vi "Generate_WayPoints_Hopping_CV.vi"(8 "NumberOfCVsAtEachPoint":i32=1, 11 "Input Cluster":T2={"Scan Rate (um/s)"=15.0, "X Start"=15.0, "X End"=15.0, "Y Start"=15.0, "Y End"=15.0, " Z Start"=15.0, "HoppingDistance"=1.0, "V"=15.0, "Z End"=15.0, "Approach Rate Hopping (um/s)"=15.0, "Retrack Rate (um/s)"=15.0, "V 2"=15.0, "Approach Rate (um/s)"=15.0, "V 3"=15.0, "CV Rate / V/s"=15.0, "V 4"=15.0, "V 1"=15.0, "HoldTime1/s"=15.0, "Hold time 2 / s"=15.0, "Hold time 3/ s"=15.0, "HoppingDistanceBetweenLines"=1.0}) -> (0 "output cluster":T1, 3 "WaitTimeScaler":u64)   [LabVIEW 2023]
uses:
  TypeDefs/WayPointCluster.ctl
  TypeDefsControls/Time.ctl
  User_Vi/Settings.vi
panel:
  in  "WayPointCluster 2":T1
  out "Y  P":dbl
  out "X  P":dbl
  out "HoppingDistanceX":dbl
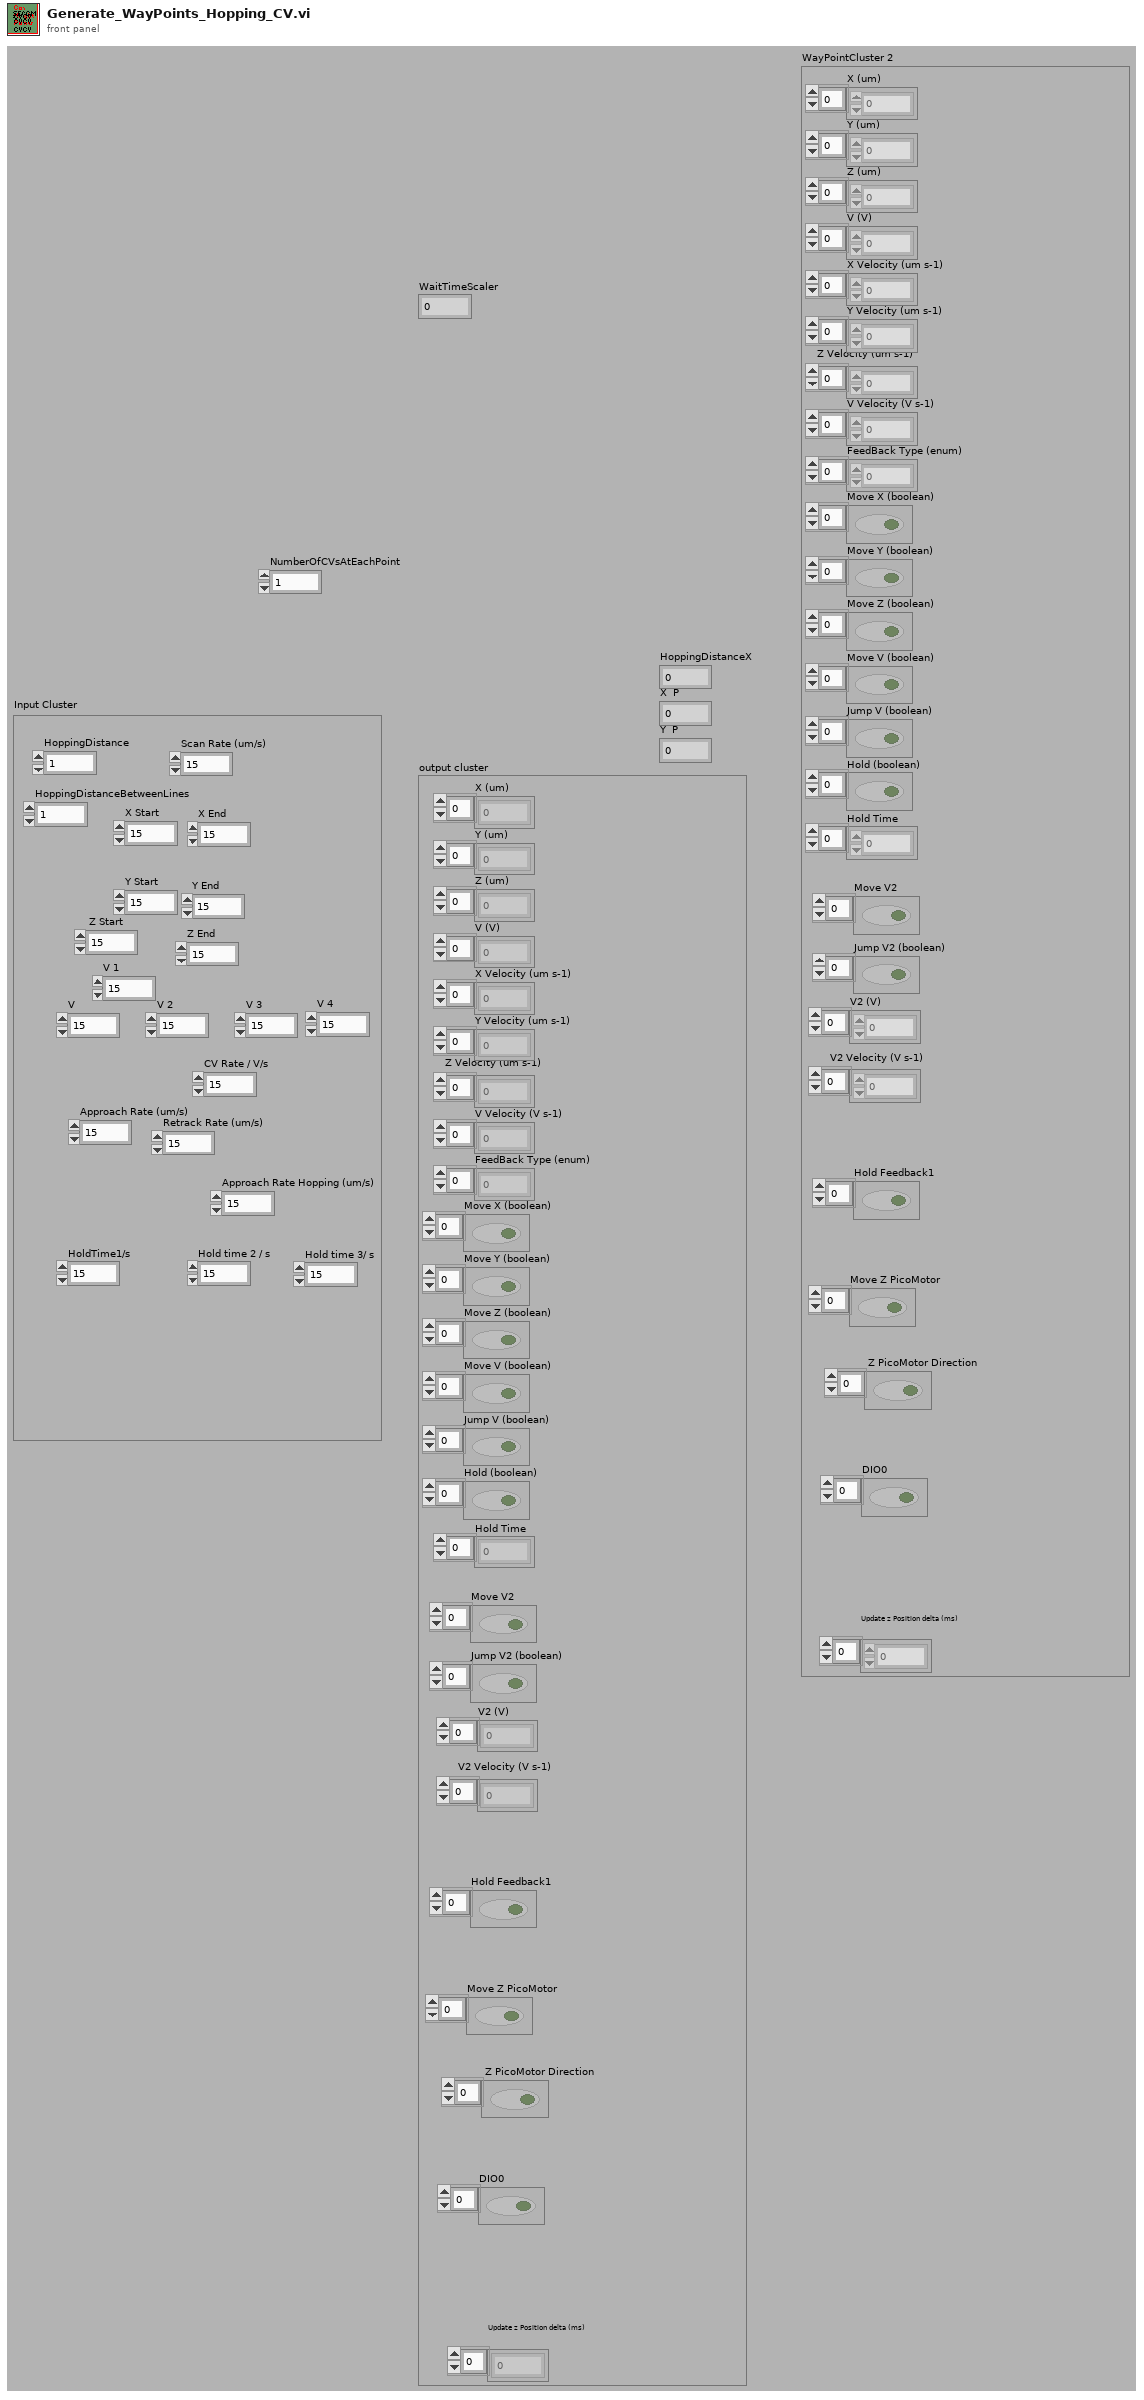
[diagram p1: front panel]
types:
  T1 = typedef "WayPointCluster.ctl" = cluster{"X (um)":dbl[], "Y (um)":dbl[], "Z (um)":dbl[], "V (V)":dbl[], "X Velocity (um s-1)":dbl[], "Y Velocity (um s-1)":dbl[], "Z Velocity (um s-1)":dbl[], "V Velocity (V s-1)":dbl[], "FeedBack Type (enum)":u16[], "Move X (boolean)":bool[], "Move Y (boolean)":bool[], "Move Z (boolean)":bool[], "Move V (boolean)":bool[], "Jump V (boolean)":bool[], "Hold (boolean)":bool[], "Hold Time":u32[], "V2 (V)":dbl[], "Move V2":bool[], "V2 Velocity (V s-1)":dbl[], "Jump V2 (boolean)":bool[], "Update z Position delta (ms)":i16[], "Hold Feedback1":bool[], "Move Z PicoMotor":bool[], " Z PicoMotor Direction":bool[], "DIO0":bool[]}
  T2 = cluster{"Scan Rate (um/s)":dbl, "X Start":dbl, "X End":dbl, "Y Start":dbl, "Y End":dbl, " Z Start":dbl, "HoppingDistance":dbl, "V":dbl, "Z End":dbl, "Approach Rate Hopping (um/s)":dbl, "Retrack Rate (um/s)":dbl, "V 2":dbl, "Approach Rate (um/s)":dbl, "V 3":dbl, "CV Rate / V/s":dbl, "V 4":dbl, "V 1":dbl, "HoldTime1/s":dbl, "Hold time 2 / s":dbl, "Hold time 3/ s":dbl, "HoppingDistanceBetweenLines":dbl}
  T3 = typedef "Time.ctl" = dbl
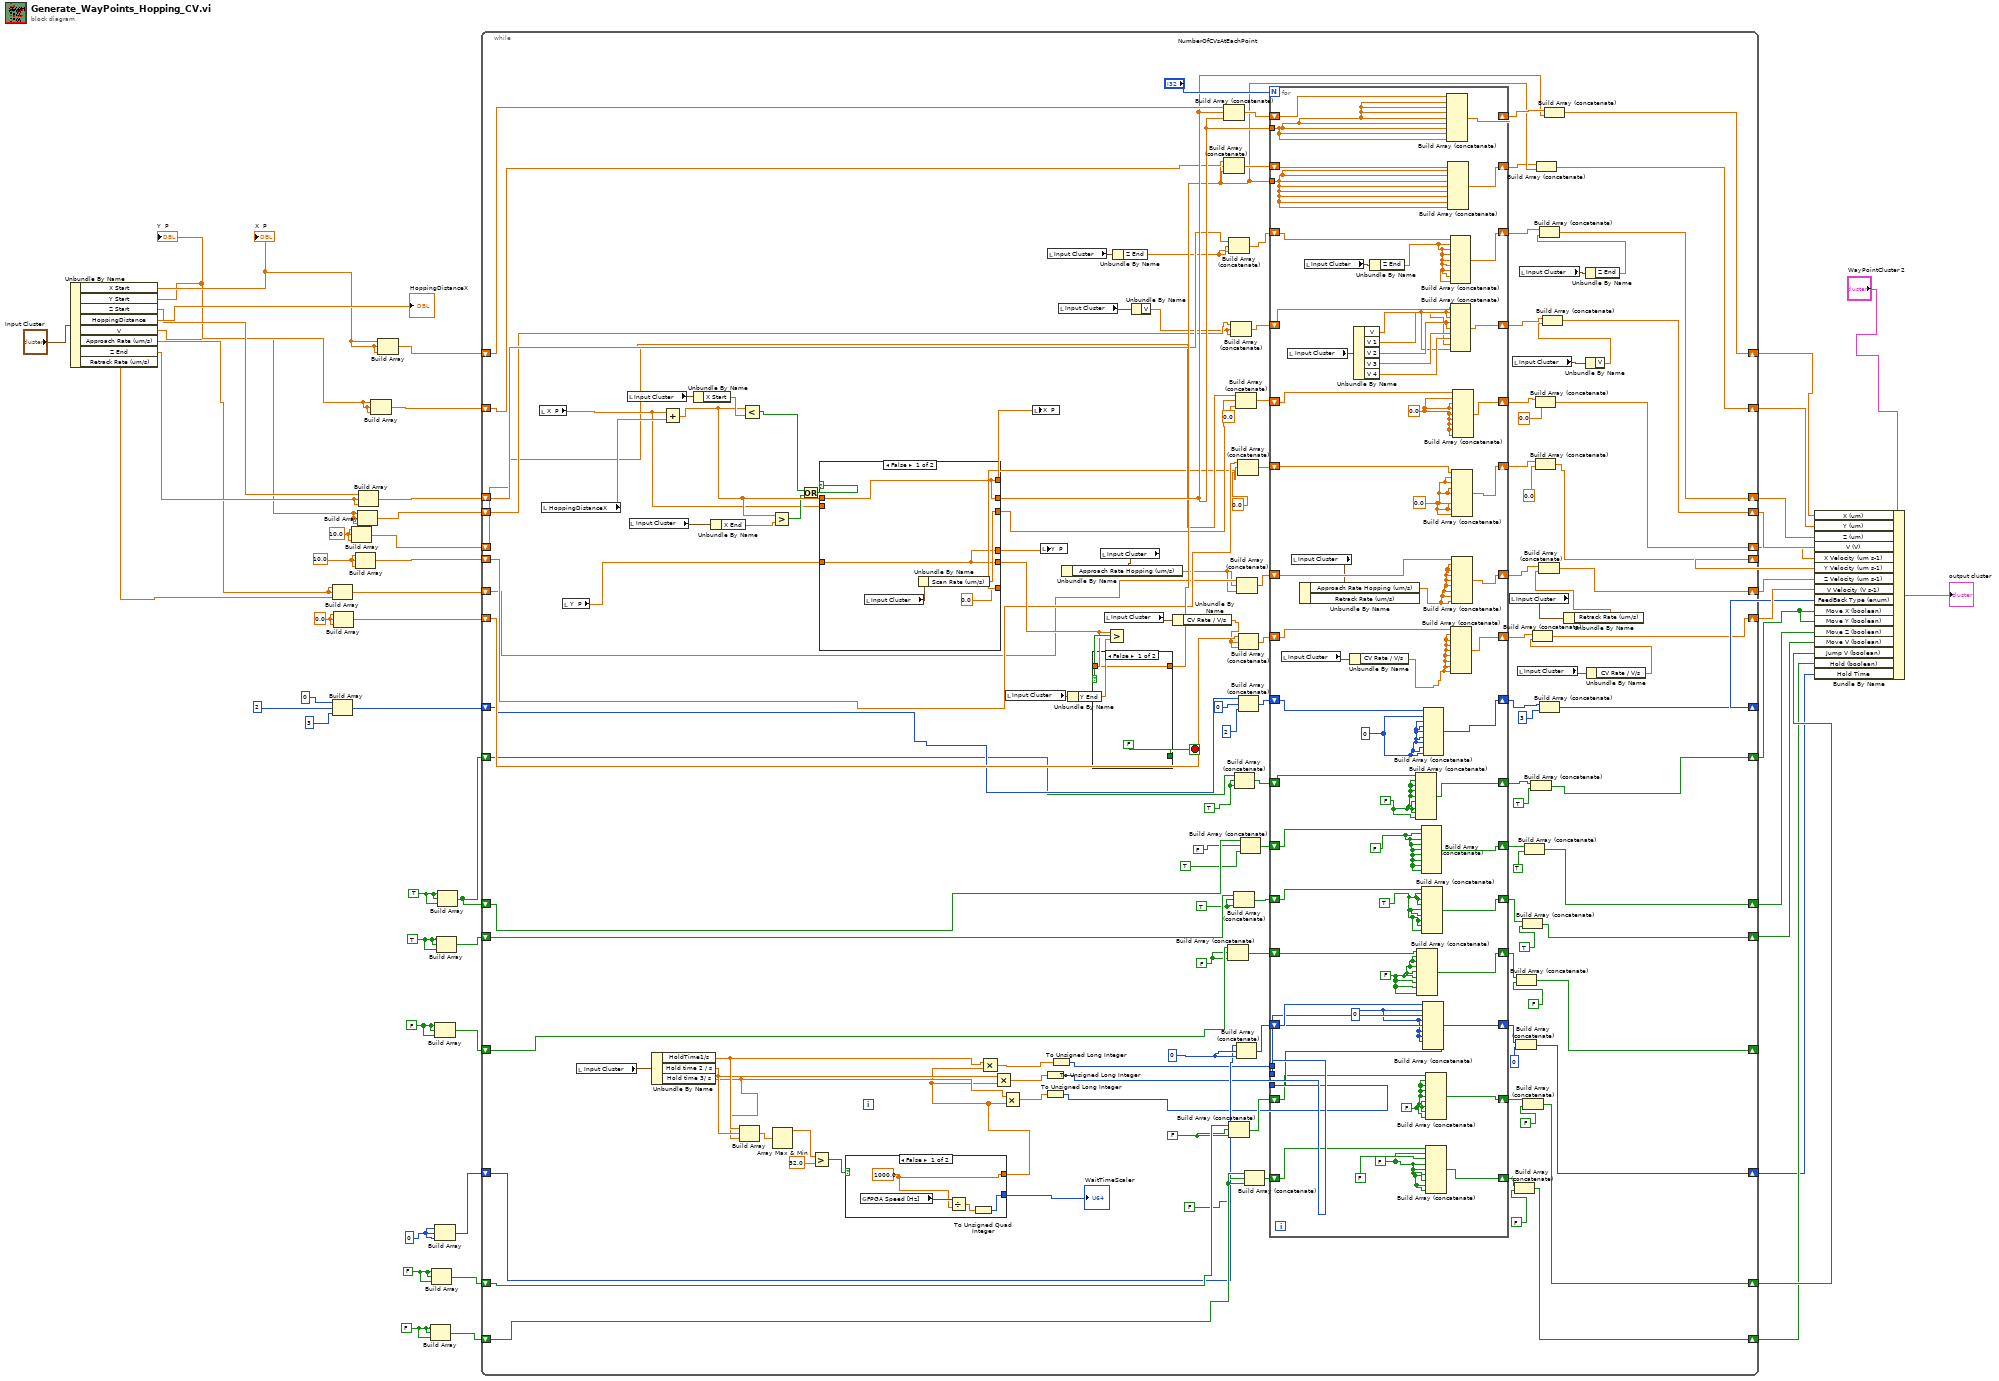
[diagram p0: block diagram]
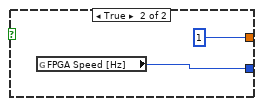
[diagram p2: hidden frame]
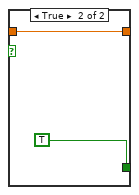
[diagram p3: hidden frame]
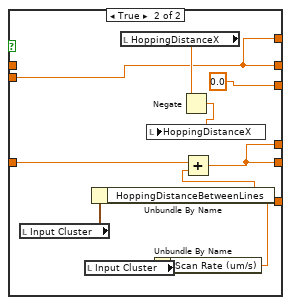
[diagram p4: hidden frame]
diagram:
  w10 = FALSE
  w18 = FALSE
  w22 = FALSE
  w21 = u32 0 ("element")
  w20 = TRUE
  w16 = TRUE
  w12 = 10.0 ("element")
  w13 = 10.0 ("element")
  w15 = 0.0 ("element")
  n1 = Unbundle By Name("Input Cluster") -> ("X Start"=w34:dbl, "Y Start"=w33:dbl, "Z Start"=w35:dbl, "HoppingDistance"=→"HoppingDistanceX":dbl, "V"=w31:dbl, "Approach Rate (um/s)"=w14:dbl, "Z End"=w32:dbl, "Retrack Rate (um/s)"=w30:dbl)
  "X  P" <- w34
  "Y  P" <- w33
  n2 = Build Array(w14, w14, w30) -> (w42:dbl[])
  n3 = Build Array(u16 0 ("element"), u16 2 ("element"), u16 3 ("element")) -> (w38:u16[])
  n4 = Build Array(w15, w15, w15) -> (w40:dbl[])
  n5 = Build Array(w12, w12, w12) -> (w45:dbl[])
  n6 = Build Array(w13, w13, w13) -> (w44:dbl[])
  n7 = Build Array(w31, w31, w31) -> (w47:dbl[])
  n8 = Build Array(w35, w32, w32) -> (w49:dbl[])
  n9 = Build Array(w33, w33, w33) -> (w50:dbl[])
  n10 = Build Array(w34, w34, w34) -> (w51:dbl[])
  n11 = Build Array(w10, w10, w10) -> (w9:bool[])
  n12 = Build Array(w22, w22, w22) -> (w26:bool[])
  n13 = Build Array(w18, w18, w18) -> (w17:bool[])
  n14 = Build Array(w21, w21, w21) -> (w4:u32[])
  n15 = Build Array(w20, w20, w20) -> (w24:bool[])
  n16 = Build Array(w16, w16, w16) -> (w11:bool[])
  n17 = while {
    shift-right: [w171] -> w6
    shift-left: w51 -> [w174]
    shift-right: [w165] -> w5
    shift-left: w50 -> [w169]
    shift-right: [w159] -> w48
    shift-left: w49 -> [w164]
    shift-right: [w155] -> w46
    shift-left: w47 -> [w153]
    shift-right: [w143] -> w28
    shift-left: w45 -> [w148]
    shift-right: [w135] -> w43
    shift-left: w44 -> [w141]
    shift-right: [w129] -> w41
    shift-left: w42 -> [w134]
    shift-right: [w120] -> w39
    shift-left: w40 -> [w126]
    shift-right: [w114] -> w37
    shift-left: w38 -> [w112]
    shift-right: [w102] -> w27
    shift-left: w11 -> [w105]
    shift-right: [w89] -> _
    shift-left: w17 -> [w92]
    shift-right: [w79] -> w25
    shift-left: w26 -> [w82]
    shift-right: [w95] -> w19
    shift-left: w24 -> [w98]
    shift-right: [w107] -> w7
    shift-left: w11 -> [w111]
    shift-right: [w75] -> w8
    shift-left: w9 -> [w78]
    shift-right: [w63] -> w3
    shift-left: w4 -> [w70]
    stop <- w182 stop-if-true
    w72 = FALSE
    w74 = FALSE
    w84 = u32 0 ("element")
    w88 = FALSE
    w93 = TRUE
    w109 = TRUE
    n18 = local read "X  P"() -> (w181:dbl)
    n19 = local read "HoppingDistanceX"() -> (w192:dbl)
    n20 = local read "Y  P"() -> (w180:dbl)
    n21 = local read "Input Cluster"() -> (w176:T2)
    n22 = local read "Input Cluster"() -> (w194:T2)
    n23 = local read "Input Cluster"() -> (w193:T2)
    n24 = Unbundle By Name(w176) -> ("HoldTime1/s"=w62:dbl, "Hold time 2 / s"=w61:dbl, "Hold time 3/ s"=w60:dbl)
    n25 = Add(x=w181, y=w192) -> (x+y=w188:dbl)
    n26 = Unbundle By Name(w194) -> ("X Start"=w191:dbl)
    n27 = Unbundle By Name(w193) -> ("X End"=w189:dbl)
    n28 = Build Array(w62, w61, w60) -> (w59:dbl[])
    n29 = Less?(x=w188, y=w191) -> (x < y?=w190:bool)
    n30 = Greater?(x=w188, y=w189) -> (0:w187:bool)
    n31 = Array Max & Min(array=w59) -> (max value=w57:dbl)  [unwired: 3 out]
    n32 = Or(x=w190, y=w187) -> (x .or. y?=w186:bool)
    n33 = Greater?(x=w57, y=T3 32.0) -> (0:w56:bool)
    n34 = case shown="False" w186 {
      tunnel: w188 -> [w265 _]
      tunnel: [w265 w271] -> w170
      tunnel: w181 -> [_ w271]
      tunnel: w180 -> [w266 w272]
      tunnel: [w266 w270] -> w179
      tunnel: [w268 0.0] -> w146
      tunnel: [0.0 w273] -> w139
      tunnel: [w266 w270] -> w178
      tunnel: [w265 w271] -> w177
      frame False {
        n35 = local read "Input Cluster"() -> (w269:T2)
        n36 = Unbundle By Name(w269) -> ("Scan Rate (um/s)"=w268:dbl)
      }
      frame True {
        n37 = local read "Input Cluster"() -> (w277:T2)
        n38 = local read "Input Cluster"() -> (w275:T2)
        n39 = Unbundle By Name(w277) -> ("HoppingDistanceBetweenLines"=w276:dbl)
        n40 = local read "HoppingDistanceX"() -> (w279:dbl)
        n41 = Unbundle By Name(w275) -> ("Scan Rate (um/s)"=w273:dbl)
        n42 = Negate(x=w279) -> (-x=w278:dbl)
        n43 = local write "HoppingDistanceX"(w278) -> ()
        n44 = Add(x=w272, y=w276) -> (x+y=w270:dbl)
      }
    }
    n45 = case shown="False" w56 {
      tunnel: [w196 w200] -> w55
      tunnel: [w195 1] -> w54
      frame False {
        w195 = 1000.0 ("y")
        n46 = global read "Settings.vi" "FPGA Speed [Hz]"() -> (w198:i64)
        n47 = Divide(x=w198, y=w195) -> (x/y=w197:dbl)
        n48 = To Unsigned Quad Integer(1:w197) -> (0:w196:u64)
      }
      frame True {
        n49 = global read "Settings.vi" "FPGA Speed [Hz]"() -> (w200:i64)
      }
    }
    "WaitTimeScaler" <- w55
    n50 = Multiply(x=w62, y=w54) -> (x*y=w69:dbl)
    n51 = Multiply(x=w61, y=w54) -> (x*y=w67:dbl)
    n52 = Multiply(x=w60, y=w54) -> (x*y=w65:dbl)
    n53 = local read "Input Cluster"() -> (w185:T2)
    n54 = local write "X  P"(w177) -> ()
    n55 = local write "Y  P"(w178) -> ()
    n56 = To Unsigned Long Integer(number=w65) -> (unsigned 32bit integer=w64:u32)
    n57 = To Unsigned Long Integer(number=w67) -> (unsigned 32bit integer=w66:u32)
    n58 = local read "Input Cluster"() -> (w163:T2)
    n59 = To Unsigned Long Integer(number=w69) -> (unsigned 32bit integer=w68:u32)
    n60 = local read "Input Cluster"() -> (w154:T2)
    n61 = Unbundle By Name(w185) -> ("Y End"=w184:dbl)
    n62 = local read "Input Cluster"() -> (w132:T2)
    n63 = Unbundle By Name(w132) -> ("Approach Rate Hopping (um/s)"=w131:dbl)
    n64 = local read "Input Cluster"() -> (w124:T2)
    n65 = Greater?(x=w179, y=w184) -> (0:w183:bool)
    n66 = case shown="False" w183 {
      tunnel: w179 -> [w262 w264]
      tunnel: [w262 w264] -> w167
      tunnel: [FALSE TRUE] -> w182
      frame False {
      }
      frame True {
      }
    }
    n67 = Unbundle By Name(w163) -> ("Z End"=w162:dbl)
    n68 = Unbundle By Name(w154) -> ("V"=w151:dbl)
    n69 = Unbundle By Name(w124) -> ("CV Rate / V/s"=w123:dbl)
    n70 = Build Array (concatenate)(w174, w170, w170) -> (w173:dbl[])
    n71 = Build Array (concatenate)(w169, w167, w167) -> (w168:dbl[])
    n72 = Build Array (concatenate)(w92, w88, w88) -> (w91:bool[])
    n73 = Build Array (concatenate)(w164, w162, w162) -> (w161:dbl[])
    n74 = Build Array (concatenate)(w82, w74, w74) -> (w81:bool[])
    n75 = Build Array (concatenate)(w153, w151, w151) -> (w152:dbl[])
    n76 = Build Array (concatenate)(w98, w93, w93) -> (w97:bool[])
    n77 = Build Array (concatenate)(w111, w109, w109) -> (w110:bool[])
    n78 = Build Array (concatenate)(w148, w146, 0.0 ("element")) -> (w147:dbl[])
    n79 = Build Array (concatenate)(w70, w84, w84) -> (w86:u32[])
    n80 = Build Array (concatenate)(w134, w131, w131) -> (w133:dbl[])
    n81 = Build Array (concatenate)(w141, w139, 0.0 ("element")) -> (w140:dbl[])
    n82 = Build Array (concatenate)(w126, w123, w123) -> (w125:dbl[])
    n83 = Build Array (concatenate)(w112, u16 0 ("element"), u16 2 ("element")) -> (w118:u16[])
    n84 = Build Array (concatenate)(w105, FALSE, TRUE) -> (w104:bool[])
    n85 = Build Array (concatenate)(w78, w72, w72) -> (w77:bool[])
    n86 = for {
      N: "NumberOfCVsAtEachPoint" -> [_]
      shift-right: [w259] -> w172
      shift-left: w173 -> [w260]
      tunnel: w170 -> [w258]
      shift-right: [w255] -> w166
      shift-left: w168 -> [w257]
      tunnel: w167 -> [w256]
      shift-right: [w251] -> w160
      shift-left: w161 -> [w254]
      shift-right: [w249] -> w156
      shift-left: w152 -> [w250]
      shift-right: [w240] -> w144
      shift-left: w147 -> [w242]
      shift-right: [w238] -> w137
      shift-left: w140 -> [w239]
      shift-right: [w235] -> w130
      shift-left: w133 -> [w236]
      shift-right: [w232] -> w121
      shift-left: w125 -> [w231]
      shift-right: [w227] -> w115
      shift-left: w118 -> [w228]
      shift-right: [w224] -> w108
      shift-left: w110 -> [w225]
      shift-right: [w221] -> w103
      shift-left: w104 -> [w222]
      shift-right: [w218] -> w96
      shift-left: w97 -> [w219]
      shift-right: [w215] -> w90
      shift-left: w91 -> [w216]
      shift-right: [w212] -> w85
      shift-left: w86 -> [w213]
      tunnel: w68 -> [w211]
      tunnel: w66 -> [w210]
      tunnel: w64 -> [w208]
      shift-right: [w206] -> w80
      shift-left: w81 -> [w207]
      shift-right: [w204] -> w76
      shift-left: w77 -> [w205]
      w201 = FALSE
      w203 = FALSE
      w209 = u32 0 ("element")
      w214 = FALSE
      w217 = TRUE
      w220 = FALSE
      w223 = FALSE
      w226 = u16 0 ("element")
      w237 = 0.0 ("element")
      w241 = 0.0 ("element")
      n87 = local read "Input Cluster"() -> (w230:T2)
      n88 = local read "Input Cluster"() -> (w248:T2)
      n89 = local read "Input Cluster"() -> (w234:T2)
      n90 = Unbundle By Name(w234) -> ("Approach Rate Hopping (um/s)"=w233:dbl)  [unwired: 1 out]
      n91 = local read "Input Cluster"() -> (w253:T2)
      n92 = Unbundle By Name(w230) -> ("CV Rate / V/s"=w229:dbl)
      n93 = Unbundle By Name(w248) -> ("V"=w243:dbl, "V 1"=w247:dbl, "V 2"=w246:dbl, "V 3"=w245:dbl, "V 4"=w244:dbl)
      n94 = Unbundle By Name(w253) -> ("Z End"=w252:dbl)
      n95 = Build Array (concatenate)(w225, w223, w223, w223, w223, w223, w223, w223, w223) -> (w224:bool[])
      n96 = Build Array (concatenate)(w216, w214, w214, w214, w214, w214, w214, w214, w214) -> (w215:bool[])
      n97 = Build Array (concatenate)(w222, w220, w220, w220, w220, w220, w220, w220, w220) -> (w221:bool[])
      n98 = Build Array (concatenate)(w219, w217, w217, w217, w217, w217, w217, w217, w217) -> (w218:bool[])
      n99 = Build Array (concatenate)(w213, w209, w211, w209, w210, w209, w209, w209, w208) -> (w212:u32[])
      n100 = Build Array (concatenate)(w228, w226, w226, w226, w226, w226, w226, w226, w226) -> (w227:u16[])
      n101 = Build Array (concatenate)(w207, w203, w203, w203, w203, w203, w203, w203, w203) -> (w206:bool[])
      n102 = Build Array (concatenate)(w205, w201, FALSE, w201, w201, w201, w201, w201, w201) -> (w204:bool[])
      n103 = Build Array (concatenate)(w260, w258, w258, w258, w258, w258, w258, w258, w258) -> (w259:dbl[])
      n104 = Build Array (concatenate)(w257, w256, w256, w256, w256, w256, w256, w256, w256) -> (w255:dbl[])
      n105 = Build Array (concatenate)(w254, w252, w252, w252, w252, w252, w252, w252, w252) -> (w251:dbl[])
      n106 = Build Array (concatenate)(w250, w247, w247, w246, w246, w245, w244, w243, w243) -> (w249:dbl[])
      n107 = Build Array (concatenate)(w231, w229, w229, w229, w229, w229, w229, w229, w229) -> (w232:dbl[])
      n108 = Build Array (concatenate)(w239, w237, w237, w237, w237, w237, w237, w237, w237) -> (w238:dbl[])
      n109 = Build Array (concatenate)(w236, w233, w233, w233, w233, w233, w233, w233, w233) -> (w235:dbl[])
      n110 = Build Array (concatenate)(w242, w241, w241, w241, w241, w241, w241, w241, w241) -> (w240:dbl[])
    }
    n111 = local read "Input Cluster"() -> (w128:T2)
    n112 = local read "Input Cluster"() -> (w150:T2)
    n113 = Build Array (concatenate)(w76, FALSE) -> (w75:bool[])
    n114 = Build Array (concatenate)(w85, u32 0 ("element")) -> (w63:u32[])
    n115 = Build Array (concatenate)(w90, FALSE) -> (w89:bool[])
    n116 = local read "Input Cluster"() -> (w122:T2)
    n117 = local read "Input Cluster"() -> (w158:T2)
    n118 = Build Array (concatenate)(w96, TRUE) -> (w95:bool[])
    n119 = Build Array (concatenate)(w80, FALSE) -> (w79:bool[])
    n120 = Build Array (concatenate)(w103, TRUE) -> (w102:bool[])
    n121 = Build Array (concatenate)(w108, TRUE) -> (w107:bool[])
    n122 = Build Array (concatenate)(w144, 0.0 ("element")) -> (w143:dbl[])
    n123 = Build Array (concatenate)(w137, 0.0 ("element")) -> (w135:dbl[])
    n124 = Build Array (concatenate)(w166, w167) -> (w165:dbl[])
    n125 = Build Array (concatenate)(w115, u16 3 ("element")) -> (w114:u16[])
    n126 = Build Array (concatenate)(w172, w170) -> (w171:dbl[])
    n127 = Unbundle By Name(w128) -> ("Retrack Rate (um/s)"=w127:dbl)
    n128 = Build Array (concatenate)(w130, w127) -> (w129:dbl[])
    n129 = Unbundle By Name(w158) -> ("Z End"=w157:dbl)
    n130 = Build Array (concatenate)(w160, w157) -> (w159:dbl[])
    n131 = Unbundle By Name(w150) -> ("V"=w149:dbl)
    n132 = Build Array (concatenate)(w156, w149) -> (w155:dbl[])
    n133 = Unbundle By Name(w122) -> ("CV Rate / V/s"=w119:dbl)
    n134 = Build Array (concatenate)(w121, w119) -> (w120:dbl[])
  }
  n135 = Bundle By Name(cluster="WayPointCluster 2", "X (um)"=w6, "Y (um)"=w5, "Z (um)"=w48, "V (V)"=w46, "X Velocity (um s-1)"=w28, "Y Velocity (um s-1)"=w43, "Z Velocity (um s-1)"=w41, "V Velocity (V s-1)"=w39, "FeedBack Type (enum)"=w37, "Move X (boolean)"=w7, "Move Y (boolean)"=w7, "Move Z (boolean)"=w27, "Move V (boolean)"=w19, "Jump V (boolean)"=w25, "Hold (boolean)"=w8, "Hold Time"=w3) -> (→"output cluster":T1)
